vi "XML to Value.vi"(8 "error in (no error)":errorcluster, 9 "Parent Name Path":string[](array[string]), 10 "Value Tree":T1, 11 "Variant in":variant) -> (0 "error out":errorcluster, 3 "Variant out":variant)   [LabVIEW 2018, in "XML Config.lvlib"]
uses:
  XML Config.lvlib
  <userlib>/_OpenG.lib/lvdata/lvdata.llb/Type Descriptor Enumeration__ogtk.ctl
panel:
  out "name path":string[](array[string])
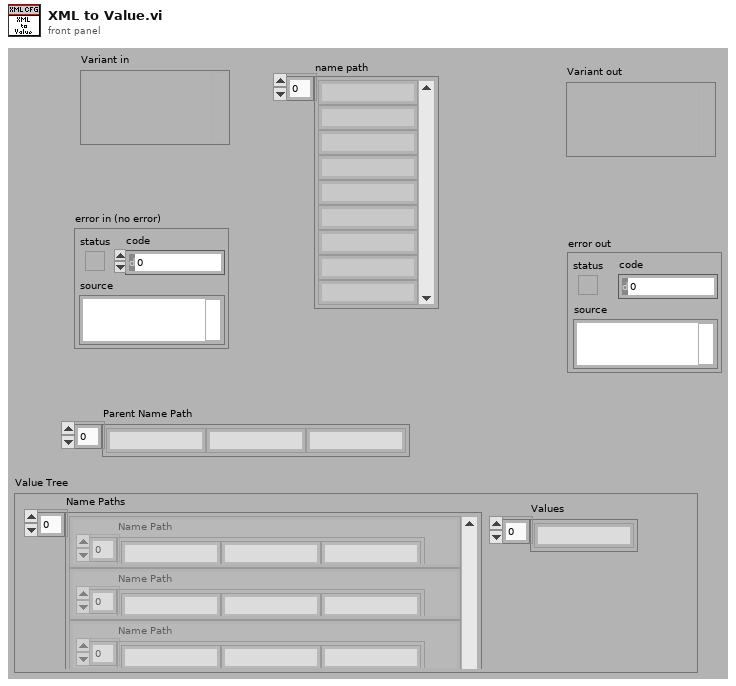
[diagram p1: front panel]
types:
  T1 = cluster{"Name Paths":cluster{"Name Path":string[]}[], "Values":string[]}
  T2 = typedef "Type Descriptor Enumeration__ogtk.ctl" = enum8{"<Null>", "I8", "I16", "I32", "I64", "U8", "U16", "U32", "U64", "SGL", "DBL", "EXT", "CSG", "CDB", "CXT", "0x0F", "0x10", "0x11", "0x12", "0x13", "0x14", "Enum U8", "Enum U16", "Enum U32", "Enum U64", "SGL PQ", "DBL PQ", "EXT PQ", "CSG PQ", "CDB PQ", "CXT PQ", "0x1F", "0x20", "Boolean", "0x22", "0x23", "0x24", "0x25", "0x26", "0x27", "0x28", "0x29", "0x2A", "0x2B", "0x2C", "0x2D", "0x2E", "0x2F", "String", "0x31", "Path", "Pict", "0x34", "0x35", "0x36", "DAQ", "0x38", "0x39", "0x3A", "0x3B", "0x3C", "0x3D", "0x3E", "0x3F", "Array", "0x41", "0x42", "0x43", "0x44", "0x45", "0x46", "0x47", "0x48", "0x49", "0x4A", "0x4B", "0x4C", "0x4D", "0x4E", "0x4F", "Cluster", "0x51", "0x52", "Variant", "Waveform", "0x55", "0x56", "0x57", "0x58", "0x59", "0x5A", "0x5B", "0x5C", "0x5D", "0x5E", "0x5F", "0x60", "0x61", "0x62", "0x63", "0x64", "0x65", "0x66", "0x67", "0x68", "0x69", "0x6A", "0x6B", "0x6C", "0x6D", "0x6E", "0x6F", "Refnum"}
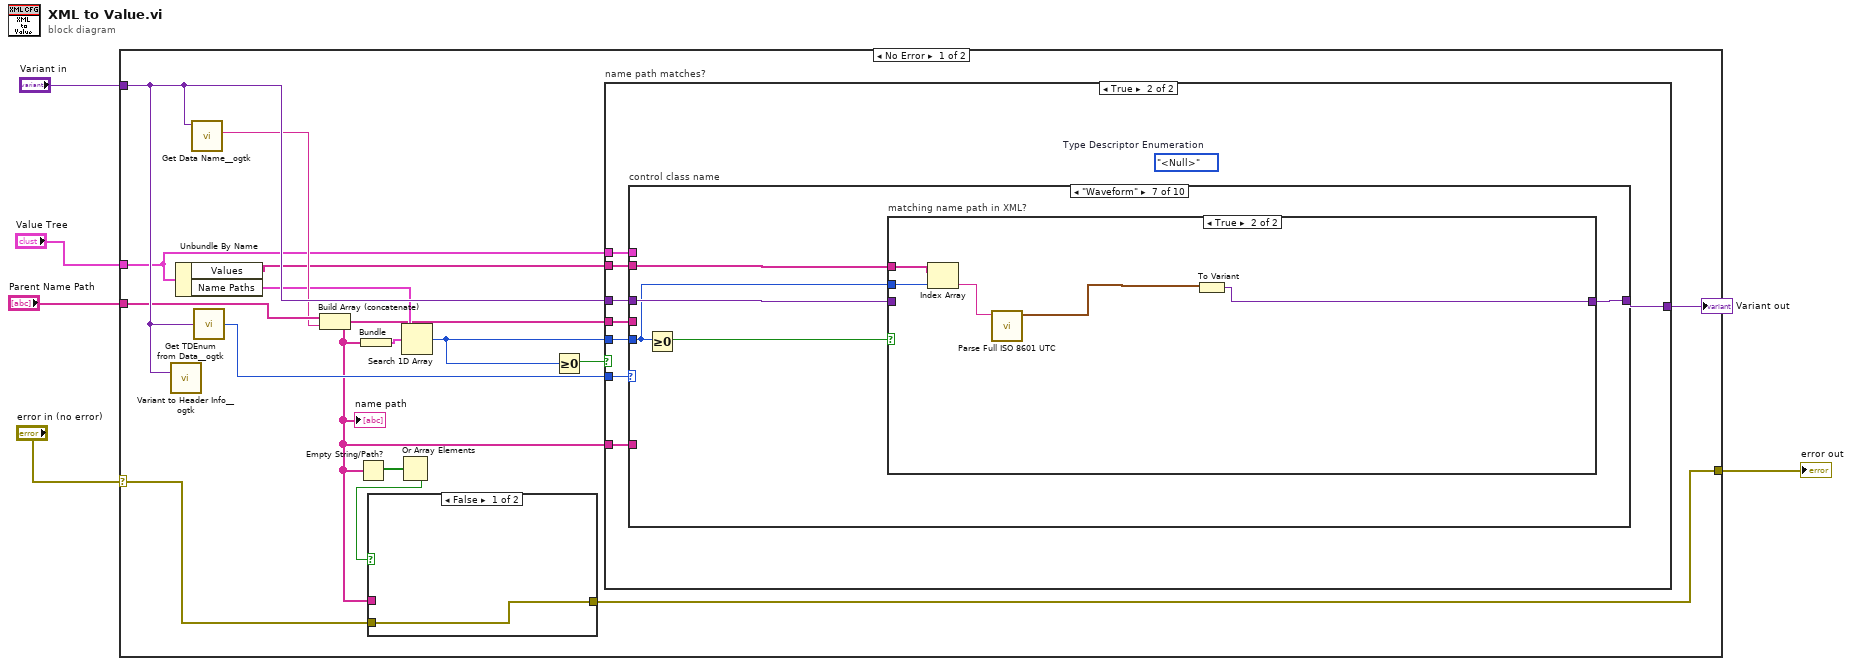
[diagram p0: block diagram]
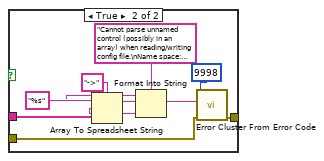
[diagram p2: hidden frame]
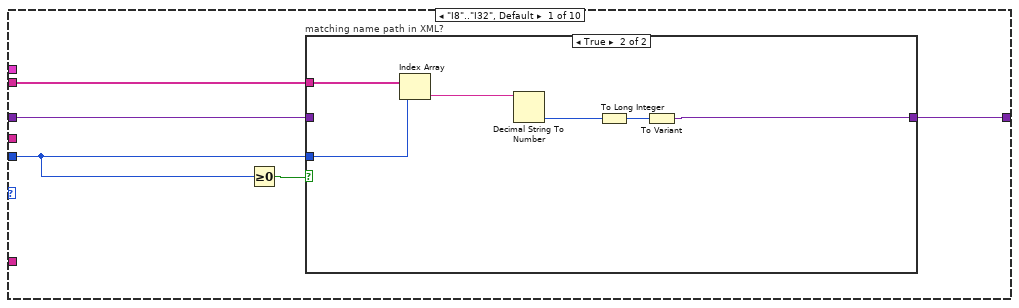
[diagram p4: hidden frame]
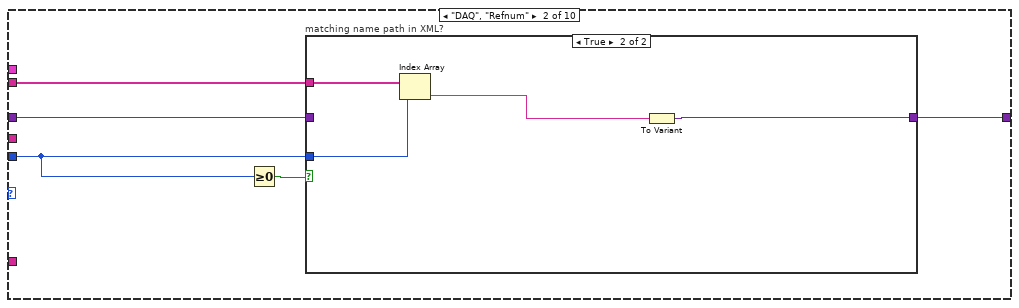
[diagram p6: hidden frame]
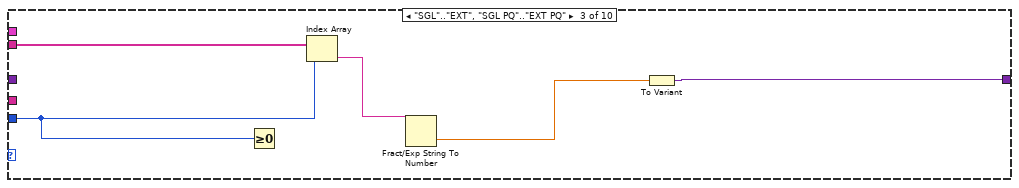
[diagram p8: hidden frame]
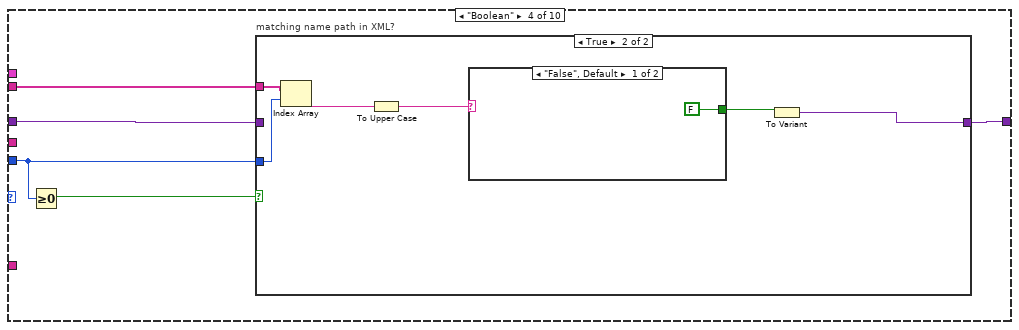
[diagram p9: hidden frame]
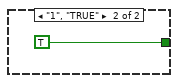
[diagram p11: hidden frame]
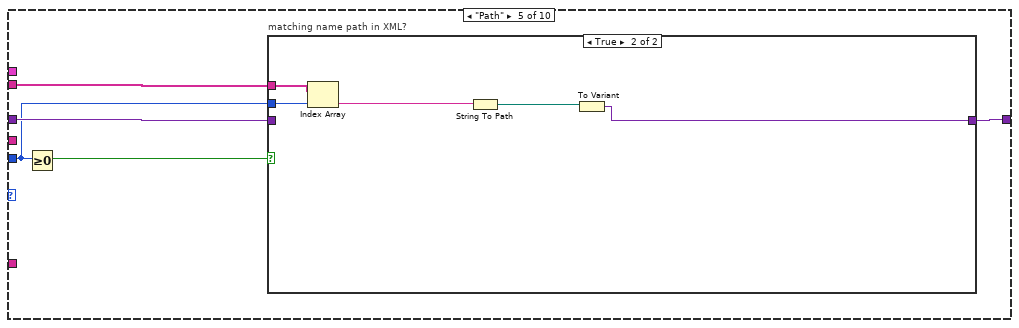
[diagram p12: hidden frame]
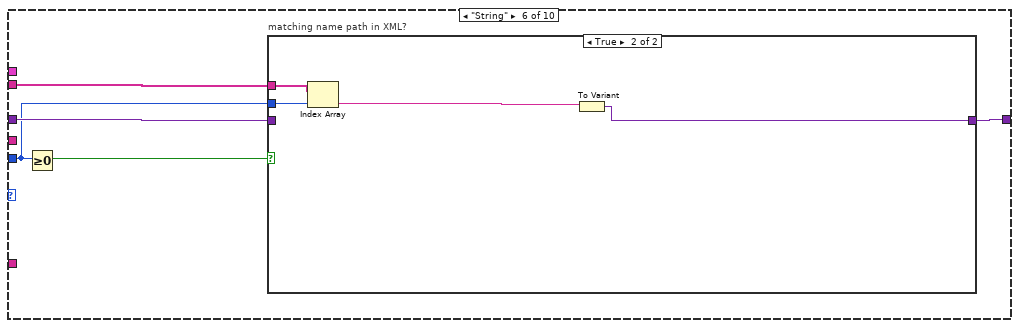
[diagram p14: hidden frame]
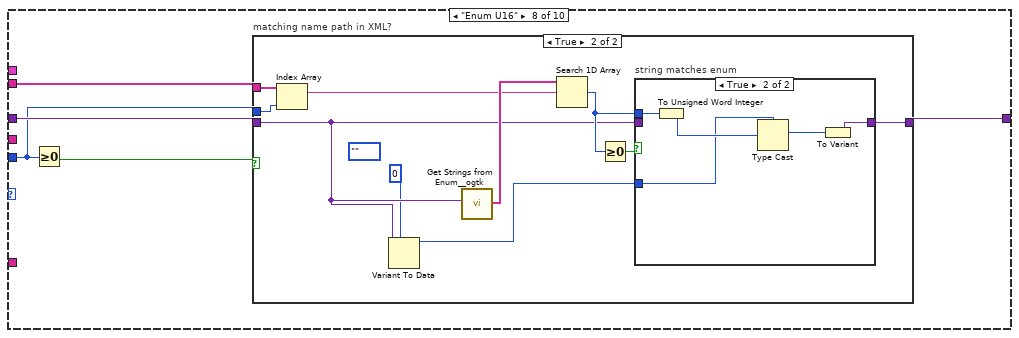
[diagram p17: hidden frame]
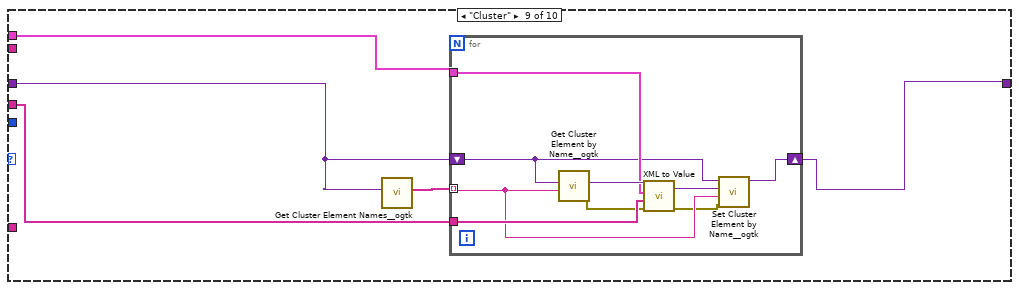
[diagram p20: hidden frame]
diagram:
  n1 = case shown="No Error" "error in (no error)" {
    selector: "error in (no error)" -> [w7 w191]
    tunnel: "Variant in" -> [w20 _]
    tunnel: "Parent Name Path" -> [w19 _]
    tunnel: "Value Tree" -> [w13 _]
    tunnel: [w6 w191] -> w1
    frame No Error {
      n2 = call <userlib>:"Variant to Header Info__ogtk.vi"("Variant"=w20) -> ()  [unwired: 3 in, 3 out]
      n3 = Unbundle By Name(w13) -> ("Values"=w15:string[], "Name Paths"=w17:cluster{"Name Path":string[]}[])
      n4 = call <userlib>:"Get Data Name__ogtk.vi"("Data"=w20) -> ("Data Name"=w18:string)  [unwired: 8 in, 2 out]
      n5 = call <userlib>:"Get TDEnum from Data__ogtk.vi"("Data"=w20) -> ("Type Descriptor Enumeration"=w21:T2)  [unwired: 4 in]
      n6 = Build Array (concatenate)(w19, w18) -> (w9:string[])
      "name path" <- w9
      n7 = Empty String/Path?(string/path=w9) -> (empty?=w10:bool[])
      n8 = Bundle(w9) -> (w16:cluster{string[]})  [unwired: 1 in]
      n9 = Or Array Elements(Boolean array=w10) -> (logical OR=w8:bool)
      n10 = case shown="False" w8 {
        tunnel: w9 -> [_ w28]
        tunnel: [w22 w24] -> w6
        tunnel: w7 -> [w22 w23]
        frame False {
        }
        frame True {
          n11 = Array To Spreadsheet String(delimiter (Tab)="->", array=w28, 3:"%s" ("format string")) -> (spreadsheet string=w29:string)
          n12 = Format Into String(format string="Cannot parse unnamed control (possibly in an array) when reading/writing config file.\nName space: %s", w29) -> (resulting string=w25:string)  [unwired: 2 in, 1 out]
          n13 = call <vilib>:"Error Cluster From Error Code.vi"("error in (no error)"=w23, "error message (\"\")"=w25, "error code (0)"=9998) -> ("error out"=w24:errorcluster)  [unwired: 6 in]
        }
      }
      n14 = Search 1D Array(1D array=w17, element=w16) -> (index of element=w12:i32)  [unwired: 1 in]
      n15 = Greater Or Equal To 0?(x=w12) -> (x >= 0?=w11:bool)
      n16 = case "name path matches?" shown="True" w11 {
        tunnel: w21 -> [_ w40]
        tunnel: w20 -> [w32 w39]
        tunnel: w15 -> [_ w38]
        tunnel: [w32 w37] -> w14
        tunnel: w9 -> [_ w36]
        tunnel: w13 -> [_ w35]
        tunnel: w12 -> [_ w34]
        tunnel: w9 -> [_ w33]
        frame False {
        }
        frame True {
          (unwired) Type_Descriptor_Enumeration__ogtk."<Null>"  # Type Descriptor Enumeration
          n17 = case "control class name" shown="\"Waveform\"" w40 {
            tunnel: w39 -> [w45 w57 _ w72 w86 w97 w107 w118 w140 w165]
            tunnel: w38 -> [w44 w56 w67 w71 w83 w94 w104 w117 _ w163]
            tunnel: w34 -> [w43 w55 w66 w69 w82 w93 w103 w115 _ w162]
            tunnel: [w41 w53 w65 w68 w84 w95 w105 w114 w138 w164] -> w37
            tunnel: w36 -> [_ _ _ _ _ _ _ _ w139 _]
            tunnel: w35 -> [_ _ _ _ _ _ _ _ w137 w157]
            tunnel: w33 -> [_ _ _ _ _ _ _ _ _ w156]
            frame "I8".."I32", Default {
              n18 = Greater Or Equal To 0?(x=w43) -> (x >= 0?=w42:bool)
              n19 = case "matching name path in XML?" shown="True" w42 {
                tunnel: w45 -> [w46 _]
                tunnel: w44 -> [_ w52]
                tunnel: w43 -> [_ w51]
                tunnel: [w46 w47] -> w41
                frame False {
                  # "No, use default value"
                }
                frame True {
                  n20 = Index Array(array=w52, index=w51) -> (element=w50:string)
                  n21 = Decimal String To Number(string=w50) -> (number=w49:i32)  [unwired: 2 in, 1 out]
                  n22 = To Long Integer(number=w49) -> (32bit integer=w48:i32)
                  n23 = To Variant(anything=w48) -> (Variant=w47:variant)
                }
              }
            }
            frame "DAQ", "Refnum" {
              n24 = Greater Or Equal To 0?(x=w55) -> (x >= 0?=w54:bool)
              n25 = case "matching name path in XML?" shown="True" w54 {
                tunnel: w57 -> [w58 _]
                tunnel: w56 -> [_ w62]
                tunnel: w55 -> [_ w61]
                tunnel: [w58 w60] -> w53
                frame False {
                  # "No, use default value"
                }
                frame True {
                  n26 = Index Array(array=w62, index=w61) -> (element=w59:string)
                  n27 = To Variant(anything=w59) -> (Variant=w60:variant)
                }
              }
            }
            frame "SGL".."EXT", "SGL PQ".."EXT PQ" {
              n28 = Greater Or Equal To 0?(x=w66) -> ()  [unwired: 1 out]
              n29 = Index Array(array=w67, index=w66) -> (element=w64:string)
              n30 = Fract/Exp String To Number(string=w64) -> (number=w63:dbl)  [unwired: 3 in, 1 out]
              n31 = To Variant(anything=w63) -> (Variant=w65:variant)
            }
            frame "Boolean" {
              n32 = Greater Or Equal To 0?(x=w69) -> (x >= 0?=w70:bool)
              n33 = case "matching name path in XML?" shown="True" w70 {
                tunnel: w72 -> [w73 _]
                tunnel: w71 -> [_ w79]
                tunnel: w69 -> [_ w78]
                tunnel: [w73 w74] -> w68
                frame False {
                }
                frame True {
                  n34 = Index Array(array=w79, index=w78) -> (element=w77:string)
                  n35 = To Upper Case(1:w77) -> (0:w76:string)
                  n36 = case shown="\"False\", Default" w76 {
                    tunnel: [FALSE TRUE] -> w75
                    frame "False", Default {
                    }
                    frame "1", "TRUE" {
                    }
                  }
                  n37 = To Variant(anything=w75) -> (Variant=w74:variant)
                }
              }
            }
            frame "Path" {
              n38 = Greater Or Equal To 0?(x=w82) -> (x >= 0?=w85:bool)
              n39 = case "matching name path in XML?" shown="True" w85 {
                tunnel: w86 -> [w87 _]
                tunnel: [w87 w88] -> w84
                tunnel: w83 -> [_ w92]
                tunnel: w82 -> [_ w91]
                frame False {
                }
                frame True {
                  n40 = Index Array(array=w92, index=w91) -> (element=w90:string)
                  n41 = String To Path(string=w90) -> (path=w89:path)
                  n42 = To Variant(anything=w89) -> (Variant=w88:variant)
                }
              }
            }
            frame "String" {
              n43 = Greater Or Equal To 0?(x=w93) -> (x >= 0?=w96:bool)
              n44 = case "matching name path in XML?" shown="True" w96 {
                tunnel: w97 -> [w98 _]
                tunnel: [w98 w100] -> w95
                tunnel: w94 -> [_ w102]
                tunnel: w93 -> [_ w101]
                frame False {
                }
                frame True {
                  n45 = Index Array(array=w102, index=w101) -> (element=w99:string)
                  n46 = To Variant(anything=w99) -> (Variant=w100:variant)
                }
              }
            }
            frame "Waveform" {
              n47 = Greater Or Equal To 0?(x=w103) -> (x >= 0?=w106:bool)
              n48 = case "matching name path in XML?" shown="True" w106 {
                tunnel: w107 -> [w108 _]
                tunnel: [w108 w111] -> w105
                tunnel: w104 -> [_ w113]
                tunnel: w103 -> [_ w112]
                frame False {
                }
                frame True {
                  n49 = Index Array(array=w113, index=w112) -> (element=w110:string)
                  n50 = call "Parse Full ISO 8601 UTC.vi"("full ISO 8601 UTC"=w110) -> ("Time Stamp"=w109:timestamp)  [unwired: 9 in, 1 out]
                  n51 = To Variant(anything=w109) -> (Variant=w111:variant)
                }
              }
            }
            frame "Enum U16" {
              n52 = Greater Or Equal To 0?(x=w115) -> (x >= 0?=w116:bool)
              n53 = case "matching name path in XML?" shown="True" w116 {
                tunnel: w118 -> [w119 w121]
                tunnel: w117 -> [_ w129]
                tunnel: w115 -> [_ w128]
                tunnel: [w119 w122] -> w114
                frame False {
                }
                frame True {
                  (unwired) enum16{""}.""
                  n54 = Index Array(array=w129, index=w128) -> (element=w126:string)
                  n55 = Variant To Data(type=u16 0 ("unsigned 16bit integer"), Variant=w121) -> (data=w123:u16)  [unwired: 1 in, 1 out]
                  n56 = call <userlib>:"Get Strings from Enum__ogtk.vi"("Enum"=w121) -> ("Enum Strings"=w127:string[])  [unwired: 7 in, 3 out]
                  n57 = Search 1D Array(1D array=w127, element=w126) -> (index of element=w125:i32)  [unwired: 1 in]
                  n58 = Greater Or Equal To 0?(x=w125) -> (x >= 0?=w124:bool)
                  n59 = case "string matches enum" shown="True" w124 {
                    tunnel: w125 -> [_ w135]
                    tunnel: w123 -> [_ w133]
                    tunnel: [w130 w131] -> w122
                    tunnel: w121 -> [w130 _]
                    frame False {
                    }
                    frame True {
                      n60 = To Unsigned Word Integer(number=w135) -> (unsigned 16bit integer=w134:u16)
                      n61 = Type Cast(type=w133, x=w134) -> (*(type *) &x=w132:u16)
                      n62 = To Variant(anything=w132) -> (Variant=w131:variant)
                    }
                  }
                }
              }
            }
            frame "Cluster" {
              n63 = call <userlib>:"Get Cluster Element Names__ogtk.vi"("Cluster"=w140) -> ("Element Names"=w136:string[])  [unwired: 9 in, 1 out]
              n64 = for {
                tunnel: w136 -> [w143] mode=indexing
                tunnel: w139 -> [w147]
                shift-right: [w145] -> w138
                shift-left: w140 -> [w146]
                tunnel: w137 -> [w148]
                n65 = call <userlib>:"Get Cluster Element by Name__ogtk.vi"("Element Name"=w143, "Cluster"=w146) -> ("error out"=w141:errorcluster, "VElement"=w149:variant)  [unwired: 7 in, 1 out]
                n66 = call "XML to Value.vi"("error in (no error)"=w141, "Parent Name Path"=w147, "Value Tree"=w148, "Variant in"=w149) -> ("error out"=w142:errorcluster, "Variant out"=w144:variant)  [unwired: 6 in]
                n67 = call <userlib>:"Set Cluster Element by Name__ogtk.vi"("error in (no error)"=w142, "Element Name (\"\": New Element Data Name)"=w143, "New Element Value"=w144, "Cluster"=w146) -> ("VCluster out"=w145:variant)  [unwired: 5 in, 2 out]
              }
            }
            frame "Array" {
              # "array dimensions\nstored in values"
              n68 = Index Array(array=w163, index=w162) -> (element=w151:string)
              n69 = String Length(string=w151) -> (length=w154:i32)
              n70 = Subtract(x=w154, y=2) -> (x-y=w152:i32)
              n71 = String Subset(string=w151, offset (0)=1, length (rest)=w152) -> (substring=w150:string)
              n72 = Spreadsheet String To Array(delimiter (Tab)=",", format string="%d", spreadsheet string=w150, array type (2D Dbl)=i32[] []) -> (array=w158:i32[])
              n73 = disable-structure shown="Enabled" {
                disable-tunnel: w165 -> [w167 w190]
                disable-tunnel: [w171 w190] -> w164
                disable-tunnel: w158 -> [w168 _]
                disable-tunnel: w157 -> [w170 _]
                disable-tunnel: w156 -> [w169 _]
                frame Enabled {
                  # "array sizes"
                  n74 = call <userlib>:"Array Size(s)__ogtk.vi"("Array"=w167) -> ()  [unwired: 8 in, 3 out]
                  n75 = call <userlib>:"Get Array Element Default Data__ogtk.vi"("Array"=w167) -> ("Array Element Default Data"=w166:variant)  [unwired: 9 in, 1 out]
                  n76 = Multiply Array Elements(1:w168) -> (0:w172:i32)
                  n77 = Greater Than 0?(x=w172) -> (x > 0?=w173:bool)
                  n78 = case shown="True" w173 {
                    tunnel: w166 -> [_ w181]
                    tunnel: w168 -> [_ w178]
                    tunnel: w172 -> [_ w180]
                    tunnel: [w174 w177] -> w171
                    tunnel: w170 -> [_ w176]
                    tunnel: w169 -> [_ w175]
                    tunnel: w167 -> [w174 _]
                    frame False {
                      # "Need to work on this to properly output a 0 element array"
                    }
                    frame True {
                      n79 = for {
                        N: w180 -> [_]
                        tunnel: w181 -> [w189]
                        tunnel: [w188] -> w179 mode=indexing
                        tunnel: w176 -> [w187]
                        tunnel: w175 -> [w183]
                        i -> [w185]
                        n80 = Format Into String(format string="element %d", w185) -> (resulting string=w184:string)  [unwired: 2 in, 1 out]
                        n81 = Build Array (concatenate)(w183, w184) -> (w182:string[])
                        n82 = call "XML to Value.vi"("Parent Name Path"=w182, "Value Tree"=w187, "Variant in"=w189) -> ("Variant out"=w188:variant)  [unwired: 7 in, 1 out]
                      }
                      n83 = call <userlib>:"Reshape 1D Array__ogtk.vi"("Size(s)"=w178, "1D Array"=w179) -> ("Reshaped VArray"=w177:variant)  [unwired: 8 in, 1 out]
                    }
                  }
                }
                frame Disabled {
                }
              }
            }
          }
        }
      }
      "Variant out" <- w14
    }
    frame Error {
    }
  }
  "error out" <- w1
